vi "PQresultStatus.vi"(8 "error in (no error)":errorcluster, 11 "res":u32) -> (0 "error out":errorcluster, 3 "PQresultStatus":T1(ring))   [LabVIEW 2018, in "libpqlv.lvlib"]
doc: "Returns the result status of the command."
uses:
  libpqlv.lvlib
  lib/libpq.dll
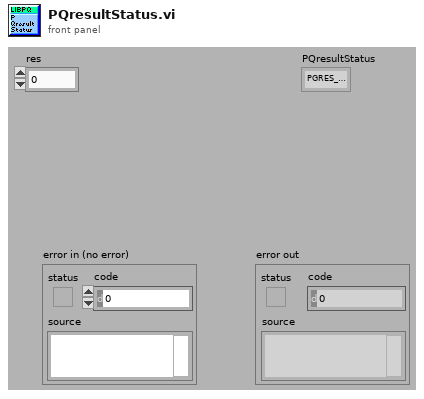
[diagram p1: front panel]
types:
  T1 = enum16{"PGRES_EMPTY_QUERY", "PGRES_COMMAND_OK", "PGRES_TUPLES_OK", "PGRES_COPY_OUT", "PGRES_COPY_IN", "PGRES_BAD_RESPONSE", "PGRES_NONFATAL_ERROR", "PGRES_FATAL_ERROR"}
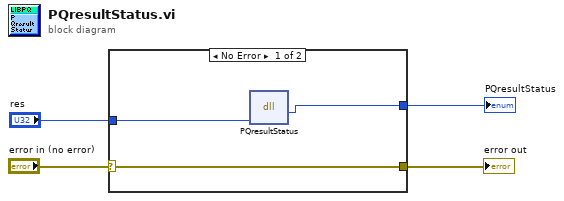
[diagram p0: block diagram]
diagram:
  n1 = case shown="No Error" "error in (no error)" {
    selector: "error in (no error)" -> [w7 w8]
    tunnel: [w7 w8] -> w3
    tunnel: [w6 _] -> w1
    tunnel: "res" -> [w5 _]
    frame No Error {
      n2 = dll-call lib="D:/Users/erics/Documents/TC-3/DAQ/PostgreSQL2LabVIEW/libpqlv/lib/libpq.*" fn="PQresultStatus"("res"=w5) -> ("PQresultStatus"=w6:u32)  [unwired: 4 in, 2 out]
    }
    frame Error {
    }
  }
  "error out" <- w3
  "PQresultStatus" <- w1
